vi "GLOBAL - FRAME END.vi"() -> ()   [LabVIEW 2017]
panel:
  out "Boolean":bool
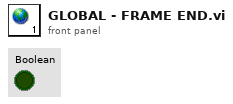
[diagram p1: front panel]
diagram:
